vi "Puzzle 13-1.vi"() -> ()   [LabVIEW 2022 SP3]
panel:
  in  "delimited string":string="LJ-L7F7..-..FLJF|JFF.-77.77-7|--F|-7F|F-7.F777FL-.FFL-L7F7-|F--F-7J-J.F-L---LF|F-J.|-FL--J-|FL-LL.|7--7-J-F-7-F|.L--77-J---77.F-7-7FF-L7F-J.\n|.|LJ|J-F-7-JL|LJLF7L7JFJJ7--.|L|J.|L-7JFFF--JF|LFF7LF7FFJF--.F-JL-7FFJ-|.LF-JJL7|-|L-JL7FF7--7|LJJL-L-7|-|F-7F--JFLL77..FF|7-.L7|L|J..FFJ..\n|.|LL7JFF7LFJ|LJ7.LJF-7FJLF-JFLF7.FL-JL-7||FLL-7.JJJ.LLJFF77.|||-7---|JL|7L|L|JF|J.7.F7JL-|..-L-7||J.J.J--|J.F-7.F7|L||7.|J-7.7.|7.LF7-FJJF7\nL-7-||77|JLJ-F|L-7.L|F|J|.|7.-7|7-JF7F.7LLJL7L-L-L.LF-7F7||F|7J.L|FJ.||F|L-|.-F-|FL|FL--LF-7.J-7F-777FFL7.LJF|F---L|7F-.FJ|J.|-L--7FF7-L7-|J\n|FJF-|-L7|.|..-JLF-||7.F-7LF-JF7J..L7.-J7FF-|..LF||-F7F|||L--77-.L|.F7-LL.-|.|L--J-|J.L7JJ-7..FLL7L7F7J.J7F--7-J7J.|L|JF7-7FJJFLJ7JJ.||L-7J7\n-77F7LLLJ|-F-|JJF|L-L77||F7|7L|LJ7F7L7..F7|LF-77FJ|L-F-J||F-7L7..JL7.F7FL-.LJ7.|JJ-JLFLJ.|FFF-7L||FJFJ-FJL7J-JFFJ.F--J--LJ|7-|FJ7|..FF7J.|77\n||7L-.||JLF|-77LF---|LFFJ.JL|F-7.FL7-777.FJ.L7L7J-JJ|L-7LJL7L-J.|..L-F7777FJ7L-|.L-|7.|L|-LJL7|.FJ|J-|-|FJJ|.LF-.-L7J.LJ|F|7.7JLL77F-JFF-L|7\nFLJJL--7F77|L--F--J-7F7|LF-FL7--.F-JFFF-LJLF7.FJJ|LFLLFJF-7L7J|7F-7J7||F7F77F77L7|7L-.FF77LF||L7L7L777.77J7||-|.F|.L7F7LLJ-JF--7L|JLLF|L-.||\nLLJ7L-L|FL7LJJ.||.|LJJL-77FJ-77J||LFL|J7|7F|-----7F7.LL-J7|FJ-F7|FJFL|LJLJL7||JLF7-|L--||L-F7L7L7L7|F7F77J--.F|7FF7LLF7-LJJFJ..-7-7|.77.L7||\n|.|L7F--7-J|LFF--7.F|FJ7|L7.|.F-7-F-F-.L|7F||.|F|.7J.LF---J|F7|||L7-LL----7|||..F-77..|LJ7-|L-JFJFJ||LJ|F7J|.-|-|||..-JFJ.FL7F|-|JFJ-|.-7|FJ\nFLJ.FLJLJ7.7F|J.|J-L-|LLJF|77FJ-FF7.|L|LJ-FF7F----7..FL---7LJLJLJFJ.FF--7FJLJ|7-L7|F--77JF7L--7|7L7LJF-J||F777J.LFL7.LLJLF7.J7L-L7|L.J7.FJJ|\n7JFFFJ7FL--F-||7|J7J..FJ.FF-F7FFFJ|77L|J-LFJ|L--7FJ-7F77F7|F-----J7F7L-7|L7F-JJF7|||F-JF-J|.F-JL7L|F-JF7|LJL77-|.||L-F|J7F7-LLJ7F-7LF-|JLLFJ\n--7F|LF7-LJ|L|77|FF.-7JJ.-FJLLFFL7|JL-JF--L7L7-FJ|-LL|L-JLJL7FF7F-7||F7|L7||F7F|||LJL7-L7FJ-L--7L-JL--JLJF7FJ-.J-JL-FJJF--JFJ|LJF|..LF-JF-77\nJ|-J--7J-F-J7|J.FF.-7|-F.L-.FLF7FJ|.-|FL77.L7L7L7|7FF|F--7F-JFJLJFJ||||L7LJLJL7|LJF--JF7|L7F7F7L-7F7F----J||-|.|-L|F-J.|||L7F|7|F7.F-LJ-7J.-\nF-J-|7LFFF7L--7F-F|--J.J..|F77|LJFJ7L77LF7FLL7|FJL7F7LJF7||F7L7F-JFJLJL7L--7F-JL-7|F7|||L7LJLJ|F-J|LJF---7LJJ.FF..L7.L7L-|-77.|JJL7.-7FF|.7.\nFJ77LJ.L7J|..L7.-J|F|77LL|-L--L-7|LF7LFFJL7FF||L-7LJL7FJ||LJL7||F7|F---JF--J|F7|FJ||L7|L7|F-7FJL-7|F7|F-7L7F7F7--|LJ77JF|JFF--JJJ.--|7FF--JJ\n.|LFLJ.|L-7-L7JL|||JL|7J.L777.F7|L7||F7L7FJF-JL7FJF-7|L7|L-7FJ|||||L7F-7L--7||L7L7||FJL7|LJFJ|F--JLJLJL7L-J|||||J.|FJ|.L-7L|.FJ7.7L7|FJ||LJ.\n-J-77F-|J.JJ.77JL7J7.LJ7-FF7F-J|L7|||||FJ|7L--7|L7L7LJFJL--JL7|LJ||FJL7|7F7|||FJFJLJ|F7|L7JL7|L7F7F----JF7FJ||L7.F-7F--FJLF|77F7-|7||J.FL--L\nFLL7JJFJ7F|F-JJ-FF77.|.FF7||L-7|FJ|||||L7L-7JFJ|FJFJF7L----7FJL-7||L-7||FJ|||||FJF--J||L7|F7|L7LJ|L---7|||L7|L7L7F--7JJ|.L--J-J--L.FL---|JJ.\n|FLJJFFL|7LJ.|.LJJL--F.L|LJL-7||L7LJ|||FJF7|FJFJL7L7|||F7F7|L7F-JLJF7LJ|L7|||||L7L-7F||FJLJ||FJF-JF---JFJ|FJ|FJFJL7FJF7F77.F|7|J|LL7.F|7J.-7\nLJ-JF|JF-|..FF|FJJ|LL|FL|F7F7LJ|FJF-J|||FJLJL7|F7|FJ||FJLJ||FJL7F--JL--J7|LJ||L7|F-JFJ|L--7|||LL-7L7F-7L7LJFJL7|F7|L7||||7.FL-JL7JL-77|-F--7\n-|F---.|FLF--J7-FFF.FFL-LJLJL7FJL7|F7|||L7|F7|||||L7||L--7|||F7||F--7F7F7L-7LJFJ|L7FJFJF7FJ||L7F-JFJ|FJFJF-JF7|||||FJ|LJL-77|.J..7.|.LJ||-|J\nLLJJ|.FL|7|..LL--||.FJL7J|LF-JL--J||LJ||FJFJLJLJLJFJ|||F-J||||LJ||F-J||||F7L-7L7|FJL7L-JLJFJ|FJ|F7L7||FJFJF7|||||LJL-JF---JF77.F.F-F77--|FJF\n|.|.L----J--.LL7.||FF77.FF-JF-7F-7LJF-J||JL----7F-JFJL7L-7LJ||F-J|L7FJLJ||L7FJFJ|L-7L----7L-JL7LJ|FJ|||FJFJ||||LJF----JFF--JL7-L7JF7||F-JL7|\nF-|77|.||L....F--7.F|L7F7L--JFJ|FJF7|F7|L7LF7F-JL-7L-7|F7L-7||L7J|FJ|F--JL7||FJL|F-J-F-7|L7F-7L7FJ|||LJL7L7LJ|L-7L7F-7F7L7F--JFLJF||J7|F7.|L\nF.L-J|7-7.L7-L|-||F7|FJ||F7F-JFJL7|LJ||L7L7|||F-7FJLFJLJ|F7||L7|FJ|FJ|F7F7|LJL7FJ|F7FJFJF7LJFJFJL7L7L7F7L-JF-JF-JFJ|FJ|L-JL---7F-7|L--JF-77.\n.|7J-JJ.-7|LFLJ-F-JLJ|7||||L--JF-JL7FJL7L7|||LJFJ|F7L--7LJ||L7|LJFJL7LJ|||L7F7||FJ||L7L7|L-7L7|F7L7L7||L7F7L7FJF-JFJL7|F------J-L|7F-|F-J.L.\n|J|7|.-L7JFFJ|F-L-7F7L-J||||F7FJF7FJL-7|FJ||L7.L7|||F7FJF-JL7|L-7L7FJF-J|L7LJ|||L7||FJFJL-7L7|LJ|-L7|LJFJ|L-JL7|F7L-7||L7F-7|L|L||FL-77JLFL|\n|7JF-J.|F-7.F|J|LFJ|L7F7LJ|FJ|L-J||F7FJLJFJ|FJF-JLJLJ|L7|F7J|L7J|FJL7|F7|FJF7||L7||LJFJF7FJFJ|F-JF7||F7L7|F-7F|LJL--JLJFJL7|J7FJL7.||LF7FF-|\nJ7-|JF-L7-7.7|||7|FJJLJL-7||FJF7FJ|||L-7FJL||LL--7F--J7||||FJFJFJL7FJLJ||L7|LJ|-||L-7|FJ|L7L-J|F7||||||FJ|L7|FJF7F--7F7L--J|JF7LF--|J7||J|LJ\n|LJJFFLLL.F-L7F-LLJJF||F-J|||F|||FJ||F7|L-7||F7F7||F7|FJ|||L7L7|F-J|F7FJL7|L-7L7||F-J|L7L-JF--J|||LJ|||L7|FJ||FJLJF7LJL7F-7L7||.L|||JF-7L-7|\nF7|.-|.|-JJJL||J|-FFF7FJF7LJ|FJLJL7|LJLJF-J|||LJ||||L7|FJ|L7L7|||F7||||F7||F7L7|||L-7L7L--7|F7FJ|L-7LJ|FJ|L7||L7F7|L--7||7L7LJL7-J7F-L.|.LF7\n.F77|J.-7JJL--F-77FFJ|L-JL7FJL--7FJL-7F7L7.||L-7||||FJ|L7|FJFJ||LJ|LJ||||||||FJ|||F7|FJF7FJLJ|L7|F-JF7|L7L-JLJFJ|LJF--J|L-7L7F7L7-F-.|-L7F7|\n|FJF|FFJL7JJLFL7|F7L7|F---J|F7F7||F7-LJL7L7||F7|||||L-JFJ|L7|FJL-7L7FJ||LJ|||L7||||||L7|||F--JFJ||F-JLJ||F---7|FJF-J-F7L--JF||L7L7J|.|.|LFF7\n.|JL.LJ--J|7FF-JLJ|F|LJF--7LJLJLJ|||F7F7L7|||||||||L-7FJ||FJ||FF7|FJL7|L7FJ||-||||||L7|||||JF7L7|||-F7F7|L--7LJ|FJLF7||FF7F7LJJ|FJJ7F|-FJFJL\nFJ7LL.F..|77LL--7FJFJF7|F-JF7F7F7LJLJ||L7||||||||||F-JL7FJ|FJL7|||L7FJL7|L7||FJLJ|||FJ||||L7||FJ||L7|||LJF-7L-7|L-7|||L-JLJL-7LLJ|.|FJLLF-7|\nFLJ.|-LF|.7JFF7FJL7L-JLJL-7|LJLJL---7||FJ|LJLJLJ|||L7F-J|FJL7FJ||L7||F-JL7||||F--J|LJ7LJ||LLJ||7LJ|LJLJF-JFJF7LJF-J||L7F-----J.LL--J-L-J|.--\nF7---7L-J-J.F|||F-J7F-7FF7LJF7F-----J||L7L7F---7LJ|FJL-7||F7||FJ|FJLJ|F-7|||LJL7F7L7JF--JL7F-JL------7FJF7L-JL-7L-7|L-JL7J.F7JF|FF7|LF.L7-||\n-F7LLL-7|F--FJLJL--7L7|FJL--J|L--7F7.|L7L7LJF7FJF-JL-7FJ|LJ|||L7|L--7LJL||LJF--J|L7L7L7F7FJL7F--7F-7FJL-JL----7|F-J|F--7L7FJL-77-|L|-7-7L.|L\n|J|-|LJ7FJF|L---7F7|FJLJF---7L7F7LJL7L7||L7FJ||||F7F-JL7|F-J|L7|L7F7L-7FJL7FJF-7|FJFJFJ||L7FJL7FJL7||F--------JLJLFJL-7L7LJF7FJJJJLF7LJL|F-7\nLLLF-L--JFFF7JF7||LJL---JFF7L7|||F--JJLJF7|L7|L7|||L--7LJ|F7|FJ|FJ|L7FJL7FJL7|FJ|L-J|L7|L7||F-JL7FJLJL--------7F-7|F--JFL--JLJF7F7.|J7F-7-L7\n|J.--F7|.F7|L7|||L7F-7F---JL7||||L---7F-J||FJ|FJLJL7F7|F-J|||L7||FJFJL7FJ|F-J|L7L--7F-J|FJ||L-7FJL7F-------7F-JL7LJL--7F7F--7FJLJL-7-F|-LJLF\nF77|LFF7FJ|L7LJ||FJL7LJF---7LJLJL---7LJF7||L7|L7|F-J|LJL7FJ|L7||LJ7L-7||FJ|F7|FJF--J|F7||FJ|F7|L7FJL------7||F7FL7F---J|||F-JL7F---JLL-7|FLF\nFFJJFJ||L7||L-7LJ|F7L--JLF7L-7F----7|F7|||L7|L7L7L-7L7F-J|L|FJLJ7F7FFJ||L7LJ||L7L--7|||||L7||||F||F7F7F---JLJ||F-JL----JLJL---JL--7J7FLJ---7\n7J.FF-JL-JL---JF7LJL77F--J|F7LJ-F--JLJ||||JLJ7L7L-7L7||F7|FJL7F--JL7L7|L7|F7||7|F-7|LJ|||FJ|||L7||||||L----7L|LJF7F-------7F7F-7F7L7LJ..7F7|\n----L-7F-7F7F7FJL7F7L7L--7LJL7F7L----7LJ|L--7F-JF7||||||||L-7LJF7F7|FJ|7LJ||LJFJL7LJFFJ|||FJ|L7||||LJ|F7JF7L-JF7||L------7LJLJ7LJ|FJJL|-|7L|\nJ-J.|.||F||||||F-J|L7|F7|L7F7LJ|F7F-7L-7|F-7|L7FJLJFJ||||L-7|F7||||||FJF--JL--JF7L--7L7|||L7|FJ|LJL-7LJ|FJL-7FJLJ|F-7F-7FJ7F----7|||---7L|LL\nJ7F-JFLJFLJ|||||F-J7||||F7LJL-7|||L7L--JLJFLJ|LJJF7L-J|||F-J||LJLJLJ|L7L---7F-7|L7F-JFLJ||FJ||FJF7F7L-7|L7F7LJLF7LJ||L7LJJFJF---JLJ-7.|L7F-L\nF77LL77F7-|LJLJLJF--JLJLJ|.F7FJLJL-JF-----------7|L---J||L-7|L-----7L-JF7F-J|FJ|FJL7F7F7LJL7|||FJLJL--JL7LJL---JL--7L-JLF7L7L-77F77|F77JLJFJ\nLJ|-LL7-|-|.F--7FL----7F7|FJLJF7F7F-JF----7F---7|L7F--7|L-7|L7F7F-7|7F-JLJF7||FJ|F7LJLJL--7LJ||L7F---7F7L---------7L---7|L-JF7L-JL--J|7...|.\nF-J.7F7|F.|FL-7|F7F---J||LJF-7|LJ||F-JF7F7LJF7FJL7||F-JL77LJFJ||L7|L7L-7F7||||L7|||F7F-7F-JF7LJ7LJJF7LJL---------7|F--7LJF7FJL7F-7F--JJJ7FJ7\n-J|FJ7JF|7|F7FJLJLJF7F7||F-JFLJFFJ||F-JLJL7FJ|L7FJLJL7F7L--7L7|L7|L-JF-J||||||FJLJ||LJFJL7FJ|F--7F7|L------7F--7FJ|L-7|F7|LJ|FJL7LJJFJ-LJ-J|\nLFJ|7F7J|.F||L7F7F7|LJLJLJF---7FJFJLJF---7||FJ-LJF-7-|||F-7|||L7LJ7F7|F7||||||L7F7|L-7L7FJ|FJL-7LJ|L-7F7F77|L-7LJLL--JLJ|L--7L7FJJ7-J7FFJLFJ\n.JFLL-JF7-FJL7||||||F--7F7|F-7LJFJJF7L7F7LJ||F7F7L7L7||LJFJL7L7L---J|||||LJ||L7||LJF7L7||FJL7F7L-7|F7LJLJL7|F7L-77F----7L7F-J|LJ7F77.7--.7J.\nF|FFJLFF7JL-7|LJLJLJL-7LJLJ|FJF-JF-JL-J||F7|LJ||L-JFJLJLFJF7L7|F7F7FJ||||F-JL7|||F-J|FJLJL-7LJL--JLJL-----J||L7FJFJF7F-J-LJLF7|F77L|-J7LFJ77\n|JL||.F||JF-JL----7F7-L7F7FJL-JF7L--7F-JLJLJF7LJF-7L--7FJFJL7|LJ|||L7LJLJL7F7||||L-7|L-77F7L7F-------7F7F7JLJJLJ-|FJLJF7.F--JL-JL-7LJ||-FJ|-\nLF7-F-FJL-JF7F7F-7LJL--J||L7F--JL---J|F---7FJL7FJFJF--JL7|F7|L7|||L7L77|F-J|LJ|||F7|L7FJFJL-J|F------J||||F--7F7FJL-7FJL-JF-------J7J-F7|.LL\nF7J7L-L-7F7|LJ||FJF7F7F-JL-JL--------JL--7|L-7LJ|L-JF7F7LJ||L7L7|L7L7L7FJF7L7FJ||||||LJ|L-7F7|L7F7F7F-JLJ|L-7LJLJF-7LJF7F7L7JF-----7.-F7J7|.\n|7LFJ|-LLJ||F-J|L7|||||F-------7F--------JL--JFF----JLJL-7||||FJL7L7L7|L7||FJ|FJLJLJF7F--7LJLJ7LJLJLJF7F7L--JF7F7L7L7FJLJL7L7|F-7F-J-7LF.LF.\nL-.L7L--J|LJL--JFLJLJLJL7F7F7F7LJF-7F77F7F-----JF7F7F7F-7||L7|L-7L7|FJ|FJ||L7|L--7F-JLJF7|F-7F7F7.F--JLJL--7FJLJ|FJFLJF77|L-J|L7LJFL.F.L77|.\nJ7LJFJ.||FF7F-7F7F7F7F7|LJ||LJL-7|FJ||FJLJF-7F7FJ|||||L7|LJFJ|F-JFJ|L7|L7||FJ|F--JL----J||L7LJLJL7L------77LJF7L|L---7|L7F7F7|FJFF7..-7L77JF\nF7JFF7FLF7||L7||LJLJLJL---J|F--7LJL-JLJF7FJLLJLJJLJ|||FJL-7L7|L-7L-J7LJ7LJ||J||F7F------J||L----7|F-----7L7F-JL7|F---J|FJ||||||F7|L7FJJ.L7.F\n||F|7J|L|LJ|L|||F7F7F-7F7F7|L-7L-------J|L-7F--7F7.||||JF-JFJ|F7L--7JJ|F7FJ|FJLJ|L7F7F7F7L7LF7F-JLJF-7F7L-J|F--S|L-7JFJL-JLJLJLJLJFJJ.FF.L7|\nLJ||JF|-L-7L-J|||LJLJ-LJLJLJF7L--------7|F7LJF7LJL7LJ|L7|F7L7LJL7F7|-LFJLJFJ|F7FJFJ|LJLJL7L-J|L7F7FJFLJL---JL--7L7FJFJF7F7F7F7F7F-J|J.|L7LL-\n..F|LJ..F7L-7FJLJF--7F7F-7F-JL---------J|||F-JL-7FJF7L7|LJ|FJ.JL||||-F|F7FJLLJ|L7L-J-F---JF-7L-J|||F-----------JLLJ.L7|LJLJLJLJLJF7F7FJ-JJ.L\nF-JJ-LF-JL--JL--7L-7||||FJL--------7F--7|||L---7|L-JL7|L7J||-JLFLJ||-LLJ||JL|.L-J7.F-JF-7FJFL-7FJ||L-----------7F7FF7||FF7F7FF7F-JLJL7JLJ-7.\n|J.|7.L7F7F7F--7|F-J|||||F7F--7F7F-J|F-J|||F---JL---7|L-JJLJ7|-L|-LJ7LJ-LJJLLFJ|F|.L--JFJ|F---J|FJ|F---7F-----7|||FJ||L7|||L-JLJF7F7FJ7..777\n7.|-7.|||LJLJF7||L-7LJ||LJ|L-7LJLJF-JL7.LJ|L------7FJL---77.J7L|||7.7.JF|JL77L7F|77FFF7L7|L---7|L7|L--7|L----7|||||FJ|FJ|||F--7FJ||LJF-7-JLJ\nLF77.--LJF---J||L-7L-7||F-JF7L7F--JF--JF7FL-7F7F7FJL--7F-J-F.7-LL77.LJFJ-..LL7LLL.-FFJL-JL7F--J|-LJ.F-JL-----JLJ|LJL-JL-JLJL-7||LLJ|FJFJJ.|7\nFJ|L7J|LLL7F-7LJF7L--JLJL-7||7LJF7.L---J|F7.LJLJLJLF-7LJJ7F--J.JJL|77L7FFF7JLL7.LF-FJF----JL7F7|F-7FJF-7F--7F77FJF7F-------7FJLJF7F7|FJJ.FL7\n7F--..JJ7.LJFJF-JL7F--7F-7LJ|F7FJL--7F--J||F------7L7L-7FJ77JFJ|FF--J-L|7F77-L7J||-L-JF7F7F7LJLJL7|L7L7LJF-J||FJFJLJF7F---7|L-7J|||||||..LJ|\n|7L|L.FFJ-LFJFJFF7LJF7||JL-7LJLJF7F7LJF7FJLJF---7FJFJF-J7L|7--|-LJJJJF|J-|F77LLJF|F-7FJLJ||L-7F7FJL7L-JF7L--J||FJF-7|||F-7|L7FJFJLJLJL7--.F7\n|J.L|-LJ|JFL7|F-JL--JLJ|F--JF7F-JLJL--JLJF--JF7LLJLL7|F777F7.L7-|...7J|F|L|L7-|7F7|FJL--7|L-7LJ|L-7|F7J|L---7LJL7L7LJ||L7|L7LJFJF7F7F7|LJ.FJ\n||FF-7.FF---J|L-----7F7|L7F7|||LF--------JF7FJL--7|FJLJL-7||JJL-J..F-JL-|-|FJFLL|LJ|F7F-JL-7L-7|F-JLJL7L---7L7F7L-JF7LJFJ|FJF7|FJLJLJLJ.F7JJ\n-7-J-L--L-7F7|F-----J|||FJ|||||FJF--------JLJF---JFJF7F-7LJ|..LLLJ-JJ..F7.||L|.FL-7||||F--7|F7||L----7L7.F7L7|||F--JL7FJFLJFJLJL----77-J-JJ7\nFF-L7FJLJLLJ|||F7F7F7|||L7|LJLJL-JF-------7F-JF7F7L7|LJF|F-J7--7JF-.|FFJ|FJ|FF7F7|||||LJF-JLJ||L----7L7L-JL-J|||L--7JLJLF-7L-7F--7F7|J7FF|7L\nF|-L--J7L|JFJ|||LJLJ||||J||F----7.L------7|L--JLJL-JL--7||J||LLF7-|-LFL7||FJFJLJL-JLJL7LL---7LJF---7L7|F-7F7L|||F-7|F7F7L7L--JL7-LJLJJ7FLJ7L\nLJ|.F|.7L-FJFJ|L7F--J|LJFJ|L7F-7L7F-----7|L7F7F7F7F----J||F-J-7.L7|-FLFJLJL7L-----7F-7L-----JF-J|F7L7LJ|-LJL7LJLJFJLJLJL-JF---7L---7JJLFJJ7|\n|7FFLJ-7J.L7L7|FJL--7|F-JFJLLJFL7|L----7LJ-LJLJLJLJF--7|LJ-L7.-7JFL77-|F-7FJ|F7|F7||FJF-7F-7FJF7FJL7L--JF---J|F77L---7F7F7L--7L7F-7|J7F7JF--\nL77FJ|FJ.L7L-JLJF7F-J|L--JF-----JL-----JF-7F---7F7FJF7L7L|.|L7LJLJFF7.LJFJ|F7||F||LJL-J-LJ-LJFJLJF7|F--7L-77F7|L7F--7LJLJ|F7FJF|L7LJ.J7L.|7.\nF|||L-JL-7L-F---JLJF-JLF7FJF-7F---------JFJ|F--J|LJFJL-JF7-JL7LLF|FJ|F-7L7LJLJL7|L7F7F---7F7FJF7FJ|LJF7L--JFJLJFJL-7L--7FJ|LJF7L-J7F7FJJ7.F|\nJ7-J||..FFLFJF7F7F-JF7FJ|L-JLLJF--------7L-JL--7L-7L----JL7-F7F777L7|L7||L-7F--JL7|||L--7||LJFJLJ|L7FJL----JF--JLF-JF--JL-JF-JL77F7|L7|.L.F-\nFJFFJFF7FJLL-JLJLJF-J|L7|F7F--7L-------7L---7F-JFFJF---7F-JFJLJ|F7-||FJL---JL77F7||||F--J|L--JF----J|F--7F-7L-7F7|F-JF7F7F7|F--JFJLJFJFF-FLJ\nLJLJFJL7JLF--7F7F7L-7L7||||L7FJ-F77F7F7L---7|L7F7L7|F7LLJF7|F--J||FJ|L-----7FJFJ||LJ|L--7L--7-L7F---JL-7LJLL7FJ|||L--J||||LJL-7.L7F-JLFJ.|-|\nF77-7JJJLFL-7LJLJ|F7L7LJLJL-JL7FJL-JLJ|F7F-J|FJ||FJLJL7F-J||L7F-J|L7L--7F7FJL7L7||F-JF7FJF-7L--J|F----7|F--7|L-J||F--7LJLJF7F7L7FJL7-|L-LJF7\nL--F||J7.F--JF7F7|||7L7F7F7F-7LJF----7||||F7LJ-|||F7F-J|F-J|FJ|F-J-L-7FJ||L-7L7||||F7|LJFJ.L-7F-JL--7FJLJF-JL7F7LJL-7L7F-7|LJL7LJF-JFJJ7.F--\n.|FL|J.77L---JLJ||||F7||||LJ7L7FJ.F--JLJLJ|L7F7||||LJF-JL7FJ|FJ|F7F--JL7||F7L7||LJLJ||F7|F---J|F-7F-JL--7|F7LLJL7F7FJFJL7|L--7|F7|LF7J.7FLF|\nF7J|L.FFF---7F--JLJLJLJ|LJ.F7FLJF7L------7L7LJLJLJL7FJF--JL7|L7|||L---7LJ||L-J||F---JLJLJL--7FJL7|L----7|LJL-7FFJ||L7|F7|L---JLJ|L7||77J|F-F\nFF7FJ-.LL--7LJF-7F-7F-7|JF7||F7FJL7F7F---JFJF--7F-7LJFJJF7F||L|||L-7F-JF-JL--7LJ|F7F7|F7F7F-J|F-JL---7FJL-7F7L7L-JL-J|||L------7L-J|L77-LJLJ\nLLJJJL|-F7LL7FJ|LJFLJL||FJLJLJ|L-7LJLJF7.FJFJF-JL7L7FJF-JL-J|FJ||F-JL-7|F7LF7|F-J|LJ|FJLJ||F7|L-7F7F7LJF-7LJL-JF7|F7-LJ|F7F----JF-7|FJF7L|.|\n-F-|FFF-J|F7LJ.F7F7F-7LJL7F7F7L--JF7F-JL-JFJFJF7FJJLJF|F----J|FJ||F7F7||||FJLJL77L7FJL7F-JLJ||F7LJLJ|F7|FJF7F7FJL-JL-77LJLJF7F--JFJ||FJ|7L7-\nLJ.|FFL7FJ||JLFJLJ|L7|LF7||LJL7F--JLJF----JFL-JLJF7LF7|L---7FJ|7|||||LJLJ|L--7FJF7|L7FJ|F-7FJ||L--7FJ|LJL-JLJLJF-----JF7F7FJLJF--JJ|LJFJ.|JJ\nFL-LF--J|FJ|F7L--7|7||FJLJL7F-J|F----JF7F7F7LF7F-J|FJ||F---JL7|FJLJ|L---7L---J|7|||FJL7LJFJL7|L--7|L-JF---7F7F7L7F7-F7||||L7F-JF---JF7L7-J.F\nFL..L--7LJFJ||.F7|L-JLJF7F7|L--JL-----JLJ||L7||L-7|L7LJL-77F7||L--7|F7F7L-7F-7L7|||L7FL7FJF7LJF7FJL7F7L--7LJ||L7LJL-JLJLJL-JL-7L7F--JL-JJ-|J\nF-F---7L7FJFJL-JLJF---7|||||F-------7F---J|FJ||F7||FJF7F-JFJ||L7FFJLJ||L-7||JL7||||FJF-JL7||F-JLJF7|||F7FJF7LJFJF-7F-7F7F-----JFJL----7J|.||\nLFL--7L-JL-JF---7FJF-7||LJLJL7F7F7F7LJF---JL7|||||||FJLJF7L7|L7L7L7F-JL7FJ||F-J|||||FJF--J||L---7||LJLJ|L-JL7JL7L7||FJ||L------JF-----JL7---\nFF-F-JF-7F7FJF--J|FJFJLJF7FF7LJLJLJL--JF-7F7||||||LJL7LFJL7|L7|FJFJ|F7FJL7||L-7LJ||||FJF7F||F7F7||L---7L----JF7L-J||L7|L7F7F7F-7L------777.|\n|L-|F-JF|||L7L--7|L7L7F7|L7||F---7F--7FJFJ|LJ|LJ|L7F-JFJF-J|FJ||FJFJ||L7FJLJJFJF-J||||L||FJ|||||LJF---JF----7|L--7|L7|L7||||||FJF7F-7F7L--7-\n7|J|||F-J|L7L7F-J|7L7||||FJ||L--7|L-7|||L-JF7L-7L7|L-7L7L-7||FJ|L7||||||L--7FJFJF-JLJL7||L7||||L-7L---7|F---J|F--JL7||FJ||||LJL7|LJ-||L-7FJJ\nLF7||-|F-J-|FJL--JF7||||||FJ|F--JL--J|L-7F7|L77L7||F-J||F-J|LJFJ-|L7||FJF--JL7||L-7F--J|L7|||||F-JJF7JLJL7.F7||F--7LJ|L7LJ|L-7FJL-7.|L7F||FF\nJ.-||FLJJ.FLJF7F7FJLJLJ|||L7|L7F7F-7|L--J||L7|F-JLJ|F-7||F7|F-J-FJFJ|LJFJF7|FJL7F-J|F7J|FJ|LJ||L77FJL7F--JFJLJLJF-JF7L-JF-JF-J|F7FJFL-J-LJF7\n.FLLJJ7|LF-F-JLJLJF7F-7LJL-JL7LJLJJL-7F7FJ|FJ|L7F--J|FJ|||||L7F7L7|LL7FJFJ|FJF-JL7FJ||FJL7L7FJ|FJFJF-JL7F-JF-7F7L--JL--7L-7L-7||||JJJ|L|FF-J\nF7J-|7F777LL-7F7F7|||FJF7F7F7L7F7F---J|||FJL7L-J|F7L|L7|||||FJ||FJL7FJL7L7|L7L7F-JL-J|L7FJFJL7||FJFJF77LJF-JFJ||F7F7F--JF-JF-JLJLJ|F777L-JLJ\nL7|7LFJ.F--FFJ|LJLJLJL-JLJLJL7|||L--7FJ||L-7L--7||L7L7||||||L7|||F7||F-JFJ|FJFJL--7F-JFJ|FJF-J||L7L-JL-7FJF7L-JLJLJ|L--7|F7L--7.FLFJ.L7.|.-J\nF|7FJ|J.|L-FJFJF----------7-FJLJL---JL7|L7FJ-F7|||FJ7||||||L7|||||LJ||F7L7|L7||FF7||F7L7|L7|F7||JL--7F-JL-JL-----7FJF7FJLJL-7FJF-.||7F|7L7J.\nF-FLJ.L--JLL-J.L---7F7F--7|FJF-7F7F-7FJL7|L7FJ|||||F7||||||FJLJ||L7FJ|||FJL7|L7FJ|||||FJ|FJ|||||F7F7|L7F7F7F7F7F-JL-JLJF7F-7LJL--J7-77L--|J7\nFJJ7|.FLJJ.|FFF7F--J|LJF-JLJFJ.LJ|L7|L-7||7||F||LJ|||||||||L7F-JL7|L7|||L-7LJFJL7LJLJ||L|L7||||||||LJFJ|||LJ||||F-----7|||FJ||.LL-JFLJJJFJ-7\nL|.F|J--777FF-JLJF-7|F-JF-7FJJF7FJFJ|F7||L7||FJL-7||||LJ|||FJ|F7FJL7|LJ|F7L-7L-7L--7FJ|FJFJ||LJLJ|L-7L7||L-7LJ|LJF7F-7LJLJL--777|L-7.F|JF|-7\nLLFJ...FJ--FJF--7|LLJL7FJFJ|F-JLJFJ7LJ||L7||||F7FJLJ|L-7LJ||FLJ|L-7||F-J||F-JF-JF7FJL-J|FJ7|L-7|FJF7|J||L7FJF-JF-JLJ.L--7F---J|J|J-|7F--J7JJ\n.F7|FFFL7JL|FJF-JL7LF7LJ-L-JL-7F7L--7FJL7||LJLJ||F7FJF7L7FLJF7FL7FJ||L7FJ|L7FJF7||L7F7FJL-7|F-JFJFJLJFJL7|L7|F7L--7F-7F7LJF77F7F7L-L7||7-L7J\nF7LL-F.L-7.LJ||F7FJFJL--------J|L-7FJL7FJ||F-7L|LJ|L7||FJF--JL--JL7|L7||FJFJ|FJLJL7||LJF7FJLJF7L7|F7FJF-J|FJ|||F7FJ|FJ|L--JL7|LJL7-|L-JJ.|L.\nFJF|F-7-|L|J-FJ||||L------7F7F7|F-JL7FJL7||L7L-JF-J|LJ|L7L7F7F7F7FJL7|LJL7|FJL--7FJ|L7FJ|L---JL7|LJ|L7|F-JL7LJLJ|L7||-|F---7LJF--J.|JL7|L-7.\n|L|-7L7L|||-|L7|LJF---7F--J|LJ||L7F-J|F7|LJ|L7F7L---7-|FJL||||LJ||F7||F--J|L7F7FJ|FJFJ|FJF-7F--J|F7L7|||F-7L---7L7LJL-JL--7|F-JLFJ7LFL-J|LFL\n|.|FJL-7.J.FJ|LJF7|F-7LJF--J7FJ|FJL7FJ||L7F--J|L7F7FJFJL7FJ||L-7|LJ|||L7F7L7||||FJ|-|FJL-J||L-7FJ|L7|||||FJF-7FJFL7F-7F7F-JLJ-F-7L-7F7J.|-.|\nJ7|LJ7-FJJ-|-F--JLJ|FJF7|F---JFJL7FJL7||FJL-7FJFLJ||LL7FJL7||F-JL7FJ|L7|||FJ||||L7|FJL---7FJF-J|FJFJ|||LJL7L7|L7F-J|FLJ||F--7FJFJJ.LF7-JJ7.J\n|J|7L-FJJFLJLL-7F-7|L7|||L-7F-JF-JL7LLJ||F7FJL-7F-J|F7LJF-J||L-7FJL7L7||||L7||||FLJL7F7F7|L7|F7||FL7|||F--JFJL-JL-7L-7-LJL7FJ|FJF7-||JJ.L-7.\n|.|JFJJ|-7.|F|.||LLJ7||LJF-JL7|L-7FJF--J||LJF7FJL-7LJL-7L7FJ|F-JL-7L7|||||FJLJLJF7F-J||||L7|||LJL-7LJLJL--7L-7F7F-JF-JF--7|L-JL7JJ.L|.--.LFL\nL7|.||FL.--L7LFJ|-F--J|F-JF-7|F--JL7L7F7|L7FJ|L-7FJF7F7|FJL7|L7F--JFJ|||||L7F---JLJF7|||L7||||F7F7L--7F---JF7LJ||F7L--JF7LJF--7|.F7LLFJ|-77J\nFL-7FL77.|7J|.L-J|L7F7|L7FJ-LJL-7F7|FJ|||FJ|FJF7|L7|||LJ|F7||FJ|F-7|FJ||||FJL--7F-7|||||FJ|||LJ|||F7FJL7F-7||F-JLJL7F7FJ|F-J.LLJ-||JJF-7F--7\n|7-JLL-F--F-JJ.L-7FLJLJ||L-7F---J|||L7||||FJL-J||FJ|||F-J|LJLJFJ|FJ|L-J||||F---J|FJ|||||L7|LJ7FJ|||LJ.FJ|.|||L--7F7LJLJFJL7L7.LJFL7L7L7JF.L7\n|J-|7|L|7-J-|.FF7JF--7F7|F7|L--7FJLJFJ|LJ|L-7F7LJL7|||L-7L7F7LL-JL7L--7LJ||L--7FJL7|||LJFJL--7L7||L--7|FJFJ|L7F7LJL---7|F7L-77|.L7L-7-L-J|.F\nL.FL-FJL-77||--7|F|F7LJLJ|LJF--J|F-7L7|F-JF7LJL--7|||L-7L7LJL7F---JF-7L-7LJF-7LJF7LJ|L-7|F7F-JFJ||F--JLJFJFJJ|||F7F7F-JLJL7FJ--J-FJJ||.|-L7L\nLLJ-LL-J|LJ7L|7.|-LJL7F7FJF-JF-7LJFJ.|||F-JL7F-7FJLJL7FJFJF-7|L7F-7L7|F7L-7L7L--JL--JF7||||L-7L7|||F----JFJF-J||||||L7.FLLLJJJJ7LJ7FJ7-|JJFJ\n.|.|7.FJ7JFJ-||FFF---J||L7L-7|L|F7|F7LJ|L7F-JL7LJ7FF-JL7L-JFJ|FJ|FJFJLJ|F-J-L7F--7F7FJ||||L7FJFJ||||F--7FJ-L-7||||||FJ7LF-J.LL---.F|.-7F77FJ\nFF.-7F7F|FFJL-|FFL7F-7||FJ-FJ|FJ||LJL7FJFJL-7FJF-7FJF7FJF--JFJ|FJL7L--7LJJF7FJ|F-J||L7||||.||-L7||||L7FJ|F7.FJ|LJLJ||F7-7L77|.|-|7|.-JLL7|J|\n7..L|77-L-J77LJ-..LJJ||LJLFJFJ|FJ|F7FJL7|F--JL-JFJL7||L7|F7FJ-||JFJF-7L--7||L7|L7FJ|FJ|||L7|L-7LJ|||FJL7LJL7L7L-7F7LJ|L---77L7|7|7L7F-.LFL-J\nLJ-FLJ-JL7L-7.|-F-FJ-LJJ||L7L7LJFJ||L7FJ||F-7F--JF-J||FJLJ|L-7LJFJFJLL7F7LJL7||FJL7|L7||L7||F-JF-J||L7FJF7FJ-|F7LJL--JF7F-J-.LF7-||LL--7.L|.\n|7..J7|7LJF-777.L-JL-.|7LJLL7|F7L7||FJL-J||FJL-7FJF7||L7F-JF7|F-JFJF-7|||F7FJLJL7FJL7|||FJ||L7|L-7|L7|L7|||F-J||F7F7F-JLJ-J|F-.L--JL|J|JFLL-\nL77..J.L-JJL|JJ..-7.L-|7..-FJ||L7||LJF---J|L7F7|L7|||L-J|F7|||L-7L-JFJLJ|||||LLFJL7FJ||||FJ|FJ-LFJ||||J|||||F7|LJ|||L7J|J7LJJJ.|7|--J.FFJ.F|\n.L--FJ7.L7|F7..|7FJFL7LFF7FL7|L7LJ|F7L7F-7|FLJ|L7LJ||||L||||LJF-JF7FJ-F-J|||-.|L7FJL7|LJLJFJL77J|FJ-LJF||LJLJ|L-7|||FJ.|.J--||.7F-J7|F|.F-7J\nF7L7-LFJJF7-JJ.LJ--|F-7L-7JF|L7L-7LJ|FJ|J|L-7FJFJ-LLJ-F-J|LJLLL7FJLJJ7L7FJLJ|FF-JL-7||JJ-L|F7L-7LJJJ.L-LJLF--JF-J||LJJ7L-FJ-J7.|F.LL7LJF7FJ7\n|JLF.L7L7L77JF7FL-FJ|-7LFF7LL-JFFJF-JL7|FJF-JL7L7JFF|.|F-JJLF7FJ|JFJJ--LJ-JJLL|F7F-JLJ.|.|||L--JJ.L7J7.FL7L7F7L7|LJ-L7J.L|J.F--F.|.||F||-J7L\n|.F7J|L7JLL-.7J-|FL|LLL-7|7L7|LLL7L7JFJ|L7L-7FJFJ-LF|-LJJL|||LJFJ.J.|F--L.|.|LLJ|L77L|-L--||JF|L7...|7FL7J|LJL7L7LJLLJFL7L7|-L-7F|J|L--J7.FL\nLJFJLJ.L-7-J7||F77-J-F|JLJ||LF77LL7|.L7|-|F7|L7|J..L|7||7FL7L7FJJ.F|---LJ7F-JLFL|FJ-.L|7||LJ.L7L|---FF7||F|J|JL7L7F-J-J7F|FF.|.F-J7L|JFF7.|.\nJFL|7-7.7L||FLFJLJ.||.|FJ-L7.JJJ.L||7LLJFJ|LJFJ|L|7|F-7LL.L7|||J7F|L||7.FLLJ||LLLJJJ7|L-|J77-LL-J|J.FF7|-JJL|LL|FJ7.FF7|7L|.FL-L-FF-|-||-LJ7\nLF7LLJ|.L.FLJ..L7J|7F|F--|.J77|F7.LJF--7L7L-7L-J.|L|JF-FJ-7LL||L|-F7L-L-7...L|.LF|7.L7.F|7FF7F|JJFFF7JL77J7.||.|L7.|7J|JLFL7LJL-L|LL777|..J7\nFL--77F7JF-7|7-JJF||LL|J7F||LFF|-7JFJF7L-JF-JJFJ---|-LJ.F.J.LLJ.LJL--|7F-|77.|7.F.|7F|-FL-7|F-L.F--.--JJJ.-7LJ-L-JJL7J.F-J|L-7|..J-7LLLJ-FJL\nLLJJF|LJ...|-L7J7.L7-LL7-F7-F-JJLLFJFJ|F-7L7JLF||F-J|7.F|-LF.L|..FLL77|77L-J-J7-F7LJFF-7--F-.|J7F|7FFJ.||FL|77F|L|.F|.|.|FJ|F.-F|7L7||JJ.|F|\nL|J.F77-F-7J||J-L7FJ7LLLJ.|LFL7F--L-J7LJ.|FJF-|||-J7FF7J|.F7--F-J77|L-J.FF77.F7JLF-LJL-|J-.|F7.JLF|JLJ7|FL.||F|LF7.-7FL7-J7LJ.FLJF.J-.|.-|-L\n.-.J.L--JL-F--JLLL|.LLL-LFJ-L.--J-.LLJJLLLJLJJFLJ7LLL-|.L-JJ.-J.LL-J7JF77LL--LJJ.7JJ--|LJJ-L7.FJLL7-|-|JJJ-LL-77L-JL|JJLLL|--.|LLL|-J-7.LLLJ"
  out "sum":i32
  out "Array":cluster{"character array":u8[][]}[](array[cluster])
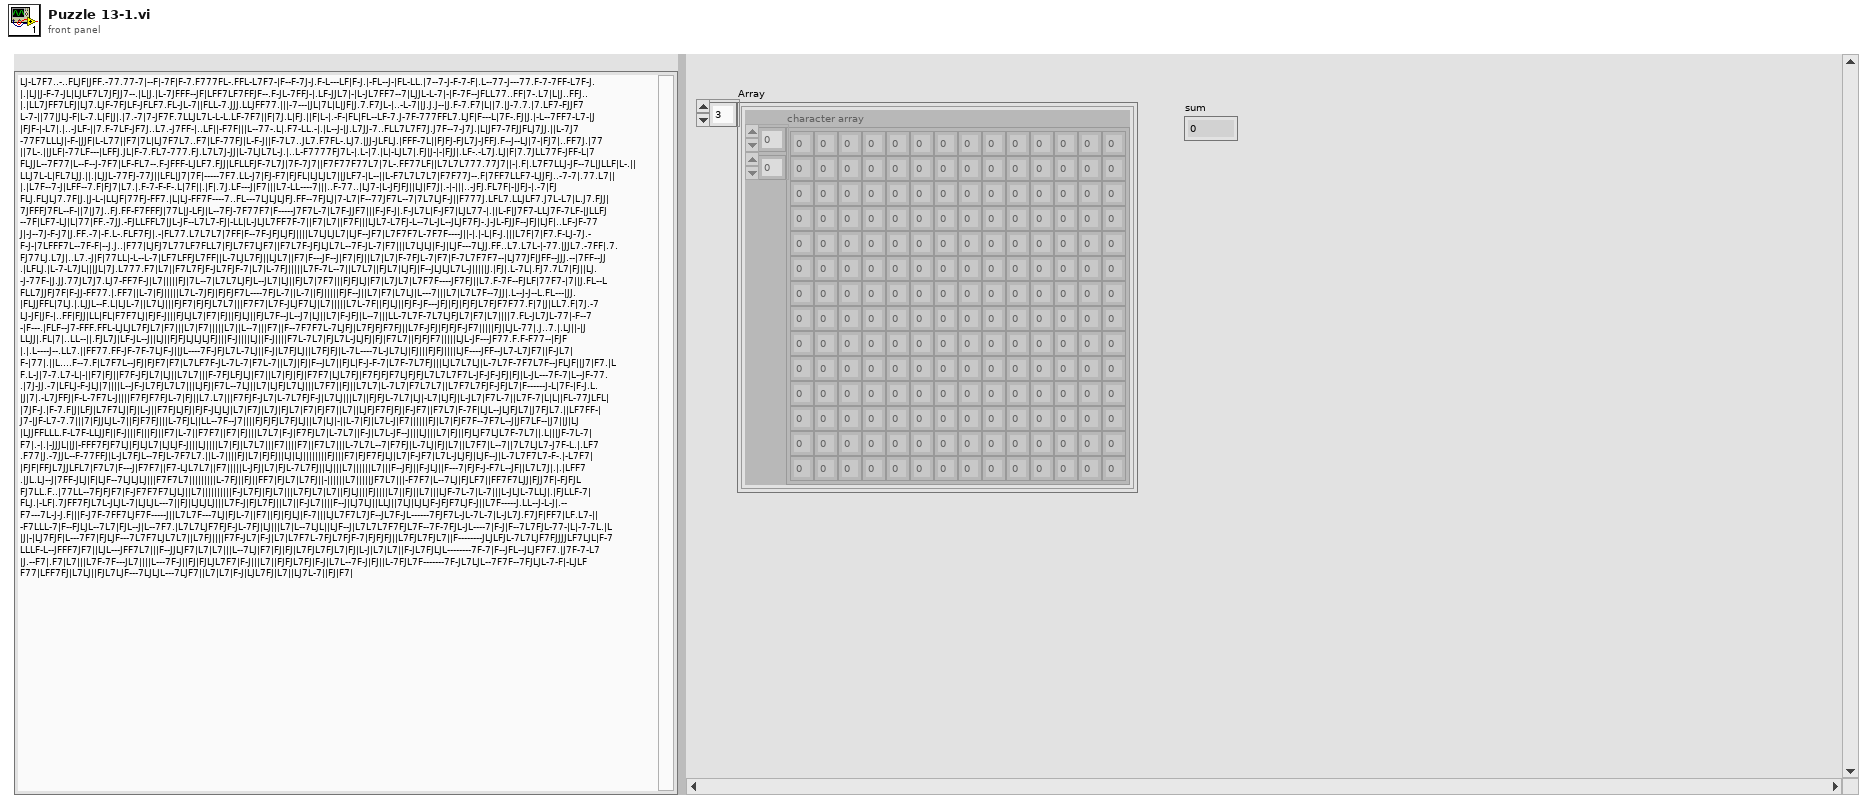
[diagram p1: front panel]
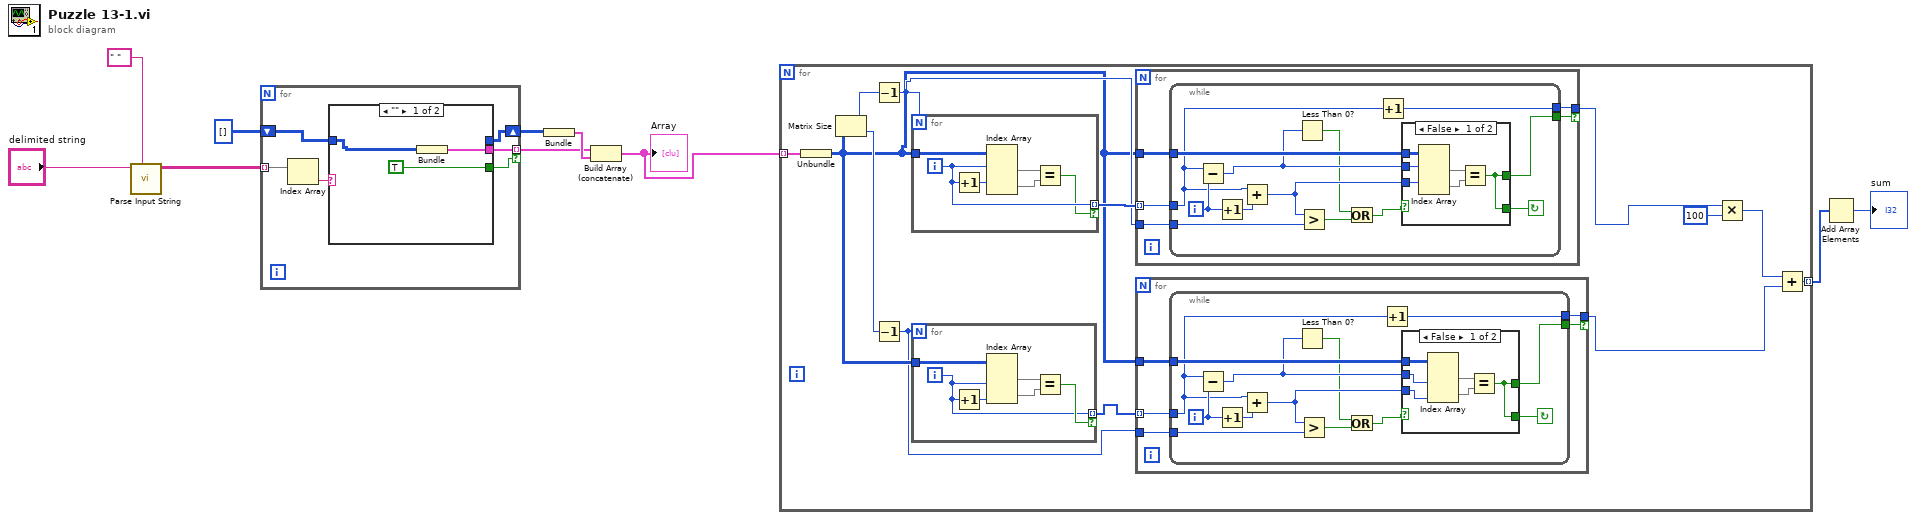
[diagram p0: block diagram]
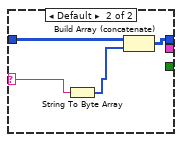
[diagram p4: hidden frame]
diagram:
  n1 = call "Parse Input String.vi"("delimiter (Tab)"=" ", "delimited string"="delimited string") -> ("parsed string"=w8:string[][])  [unwired: 9 in]
  n2 = for {
    tunnel: w8 -> [w16] mode=indexing
    shift-right: [w13] -> w6
    shift-left: u8[][] [] ("character array") -> [w14]
    tunnel: [w12] -> w4 mode=indexing if=w11
    n3 = Index Array(array=w16) -> (element=w15:string)  [unwired: 1 in]
    n4 = case shown="\"\"" w15 {
      selector: w15 -> [_ w21]
      tunnel: w14 -> [w19 w23]
      tunnel: [_ w22] -> w13
      tunnel: [w18 _] -> w12
      tunnel: [TRUE _] -> w11
      frame "" {
        n5 = Bundle("character array"=w19) -> (w18:cluster{"character array":u8[][]})  [unwired: 1 in]
      }
      frame Default {
        n6 = String To Byte Array(string=w21) -> (unsigned byte array=w20:u8[])
        n7 = Build Array (concatenate)(w23, w20) -> (w22:u8[][])
      }
    }
  }
  n8 = Bundle("character array"=w6) -> (w5:cluster{"character array":u8[][]})  [unwired: 1 in]
  n9 = Build Array (concatenate)(w4, w5) -> (w3:cluster{"character array":u8[][]}[])
  "Array" <- w3
  n10 = for {
    tunnel: w3 -> [w36] mode=indexing
    tunnel: [w31] -> w2 mode=indexing
    n11 = Unbundle(w36) -> ("character array"=w27:u8[][])
    n12 = Matrix Size(0:w27) -> (1:w35:i32, 2:w34:i32)
    n13 = Decrement(x=w35) -> (x-1=w29:i32)
    n14 = Decrement(x=w34) -> (x-1=w25:i32)
    n15 = for {
      N: w29 -> [_]
      tunnel: w27 -> [w98]
      tunnel: [w94] -> w30 mode=indexing if=w93
      i -> [w94]
      n16 = Increment(x=w94) -> (x+1=w97:i32)
      n17 = Index Array(array=w98, index (row) #1=w94, index (row) #2=w97) -> (element #1=w96:u8[], element #2=w95:u8[])  [unwired: 2 in]
      n18 = Equal?(x=w96, y=w95) -> (x = y?=w93:bool)
    }
    n19 = for {
      N: w25 -> [_]
      tunnel: w27 -> [w92]
      tunnel: [w87] -> w26 mode=indexing if=w89
      i -> [w87]
      n20 = Increment(x=w87) -> (x+1=w88:i32)
      n21 = Index Array(array=w92, index (col) #1=w87, index (col) #2=w88) -> (element #1=w91:u8[], element #2=w90:u8[])  [unwired: 2 in]
      n22 = Equal?(x=w91, y=w90) -> (x = y?=w89:bool)
    }
    n23 = for {
      tunnel: w30 -> [w66] mode=indexing
      tunnel: w27 -> [w65]
      tunnel: w29 -> [w64]
      tunnel: [w63] -> w28 if=w62
      n24 = while {
        tunnel: w66 -> [w73]
        tunnel: w65 -> [w79]
        tunnel: w64 -> [w74]
        tunnel: [w67] -> w63 if=w68
        tunnel: [w68] -> w62
        i -> [w78]
        stop <- w69 continue-if-true
        n25 = Subtract(x=w73, y=w78) -> (x-y=w76:i32)
        n26 = Increment(x=w78) -> (x+1=w77:i32)
        n27 = Add(x=w73, y=w77) -> (x+y=w75:i32)
        n28 = Less Than 0?(x=w76) -> (x < 0?=w72:bool)
        n29 = Greater?(x=w75, y=w74) -> (0:w71:bool)
        n30 = Or(x=w72, y=w71) -> (x .or. y?=w70:bool)
        n31 = Increment(x=w73) -> (x+1=w67:i32)
        n32 = case shown="False" w70 {
          selector: w70 -> [_ w86]
          tunnel: w79 -> [w85 _]
          tunnel: w76 -> [w82 _]
          tunnel: w75 -> [w81 _]
          tunnel: [w80 w86] -> w68
          tunnel: [w80 _] -> w69
          frame False {
            n33 = Index Array(array=w85, index (row) #1=w82, index (row) #2=w81) -> (element #1=w84:u8[], element #2=w83:u8[])  [unwired: 2 in]
            n34 = Equal?(x=w84, y=w83) -> (x = y?=w80:bool)
          }
          frame True {
          }
        }
      }
    }
    n35 = for {
      tunnel: w26 -> [w41] mode=indexing
      tunnel: w27 -> [w40]
      tunnel: w25 -> [w39]
      tunnel: [w38] -> w32 if=w37
      n36 = while {
        tunnel: w41 -> [w48]
        tunnel: w40 -> [w54]
        tunnel: w39 -> [w49]
        tunnel: [w42] -> w38 if=w43
        tunnel: [w43] -> w37
        i -> [w53]
        stop <- w44 continue-if-true
        n37 = Subtract(x=w48, y=w53) -> (x-y=w51:i32)
        n38 = Increment(x=w53) -> (x+1=w52:i32)
        n39 = Add(x=w48, y=w52) -> (x+y=w50:i32)
        n40 = Less Than 0?(x=w51) -> (x < 0?=w47:bool)
        n41 = Greater?(x=w50, y=w49) -> (0:w46:bool)
        n42 = Or(x=w47, y=w46) -> (x .or. y?=w45:bool)
        n43 = Increment(x=w48) -> (x+1=w42:i32)
        n44 = case shown="False" w45 {
          selector: w45 -> [_ w61]
          tunnel: w54 -> [w60 _]
          tunnel: w51 -> [w56 _]
          tunnel: w50 -> [w55 _]
          tunnel: [w57 w61] -> w43
          tunnel: [w57 _] -> w44
          frame False {
            n45 = Index Array(array=w60, index (col) #1=w56, index (col) #2=w55) -> (element #1=w59:u8[], element #2=w58:u8[])  [unwired: 2 in]
            n46 = Equal?(x=w59, y=w58) -> (x = y?=w57:bool)
          }
          frame True {
          }
        }
      }
    }
    n47 = Multiply(x=w28, y=100) -> (x*y=w33:i32)
    n48 = Add(x=w33, y=w32) -> (x+y=w31:i32)
  }
  n49 = Add Array Elements(numeric array=w2) -> (sum=→"sum":i32)
